vi "Draw Tree Elements.vi"(0 "Decision Tree In":T3, 1 "[user-specified font]":T2, 2 "Width Padding":i32, 3 "Height Padding":i32, 5 "2D Picture in":picture, 7 "Outcome Font":T2, 9 "pen":T1, 11 "Leaf Circle Radius":i32=8) -> (4 "2D Picture out":picture)   [LabVIEW 2025]
uses:
  Types/Decision Tree.ctl
  Types/Sequencing Tree Node.ctl
  Types/Single Cmd Info.ctl
  <vilib>/picture/picture.llb/imagedata.ctl
  <vilib>/Analysis/baseanly.llb/Mean (DBL).vi
  <vilib>/Analysis/NI_AALBase.lvlib
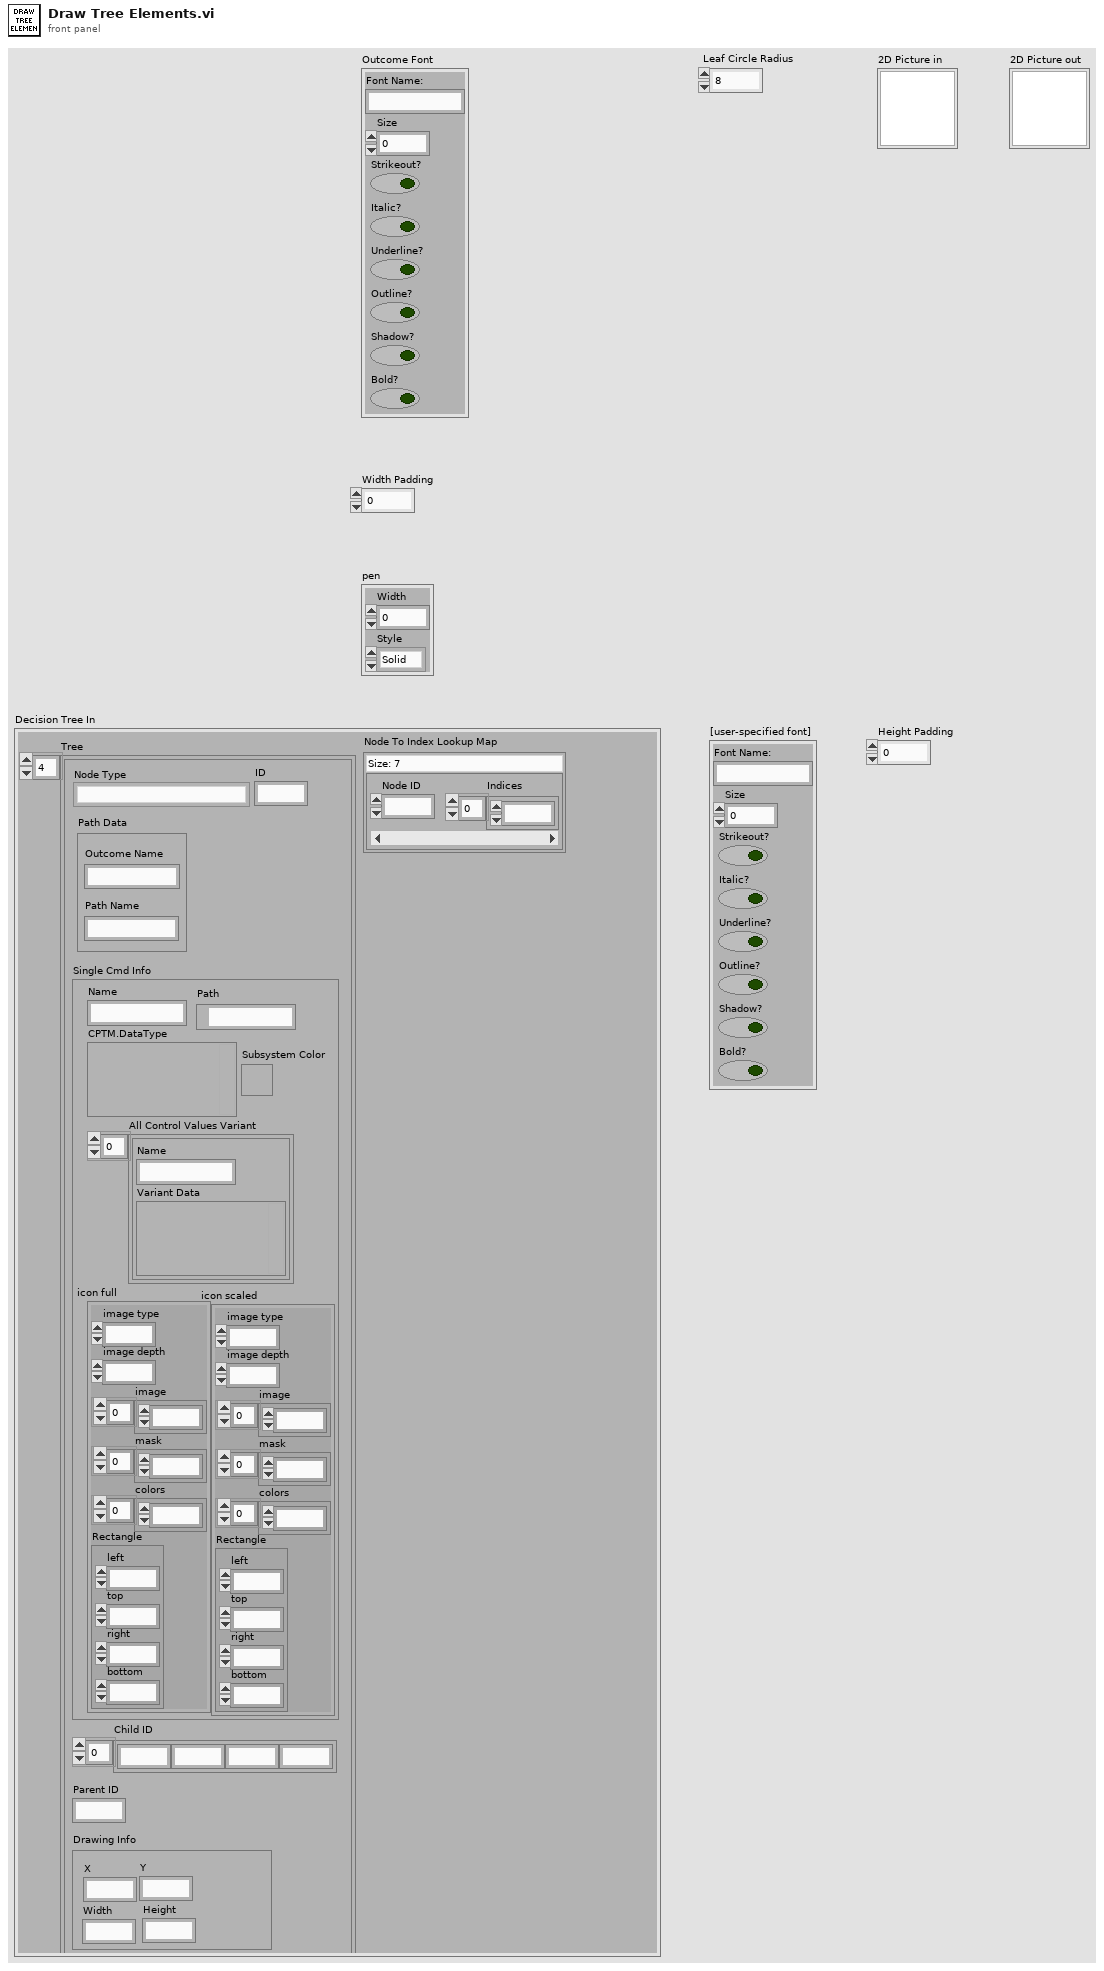
[diagram p1: front panel]
types:
  T1 = cluster{"Width":i16, "Style":enum32{"Solid", "Dash", "Dot", "DashDot", "DashDotDot"}}
  T2 = cluster{"Font Name:":string, "Size":i16, "Strikeout?":bool, "Italic?":bool, "Underline?":bool, "Outline?":bool, "Shadow?":bool, "Bold?":bool}
  T3 = typedef "Decision Tree.ctl" = cluster{"Tree":T4[], "Node To Index Lookup Map":map{i16, i16[]}}
  T4 = typedef "Sequencing Tree Node.ctl" = cluster{"Node Type":enum16{"Path", "Command", "Leaf"}, "ID":i16, "Path Data":cluster{"Path Name":string, "Outcome Name":string}, "Single Cmd Info":T5, "Child ID":i32[], "Parent ID":i32, "Drawing Info":cluster{"X":i32, "Y":i32, "Width":i32, "Height":i32}}
  T5 = typedef "Single Cmd Info.ctl" = cluster{"Name":string, "CPTM.DataType":variant, "All Control Values Variant":cluster{"Name":string, "Variant Data":variant}[], "icon full":T6, "icon scaled":T6, "Path":path, "Subsystem Color":u32}
  T6 = typedef "imagedata.ctl" = cluster{"image type":i32, "image depth":i32, "image":u8[], "mask":u8[], "colors":u32[], "Rectangle":cluster{"left":i16, "top":i16, "right":i16, "bottom":i16}}
  T7 = cluster{"Width":u16, "Style":enum32{"Solid", "Dash", "Dot", "DashDot", "DashDotDot"}}
  T8 = cluster{"horizontal":enum16{"left", "center", "right"}, "vertical":enum16{"top", "center", "bottom"}}
  T9 = enum16{"User-specified Font", "Application Font", "System Font", "Dialog Font"}
  T10 = cluster{"Path Name":string, "Outcome Name":string}
  T11 = cluster{"X":i32, "Y":i32, "Width":i32, "Height":i32}
  T12 = cluster{"left":i16, "top":i16, "right":i16, "bottom":i16}
  T13 = cluster{"[0]":dbl, "[1]":dbl, "[2]":dbl, "[3]":dbl}
  T14 = cluster{"X":dbl, "Y":dbl, "Width":dbl, "Height":dbl}
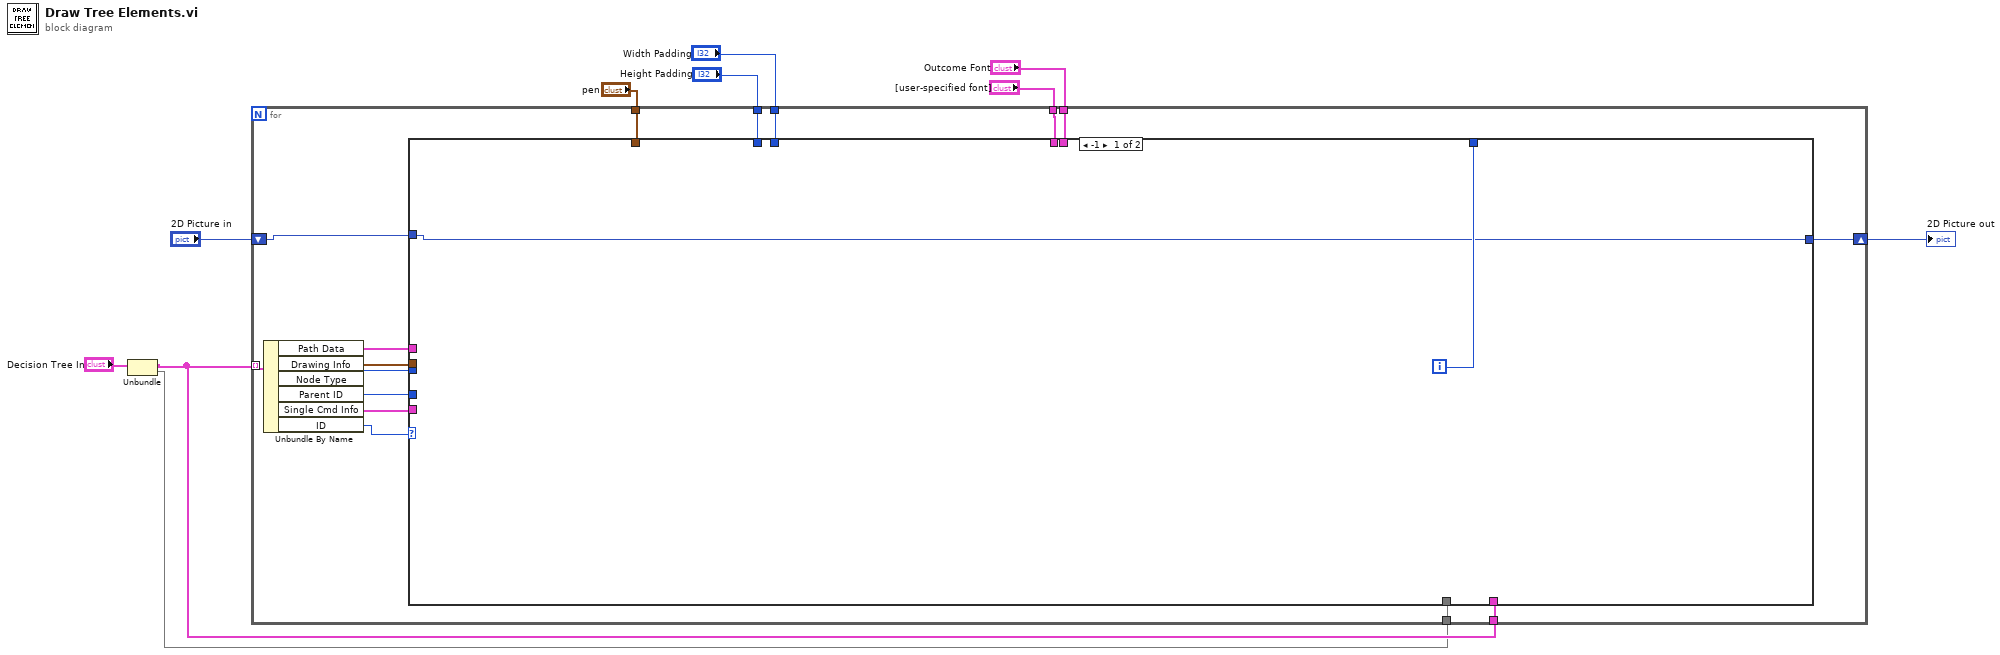
[diagram p0: block diagram]
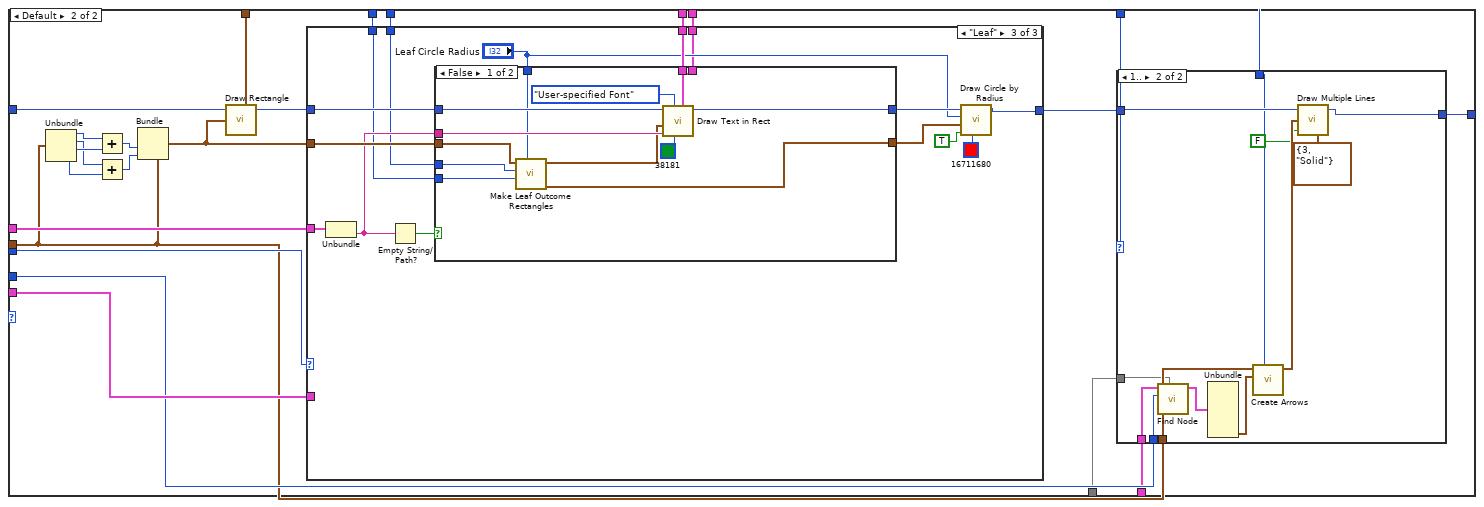
[diagram p2: hidden frame]
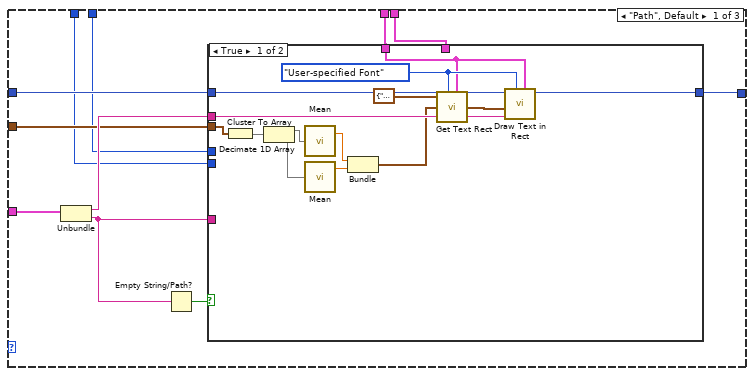
[diagram p4: hidden frame]
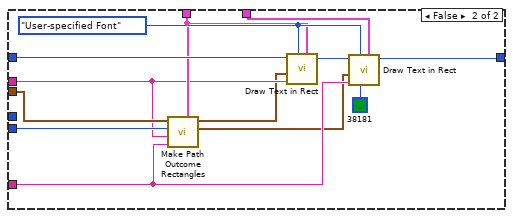
[diagram p5: hidden frame]
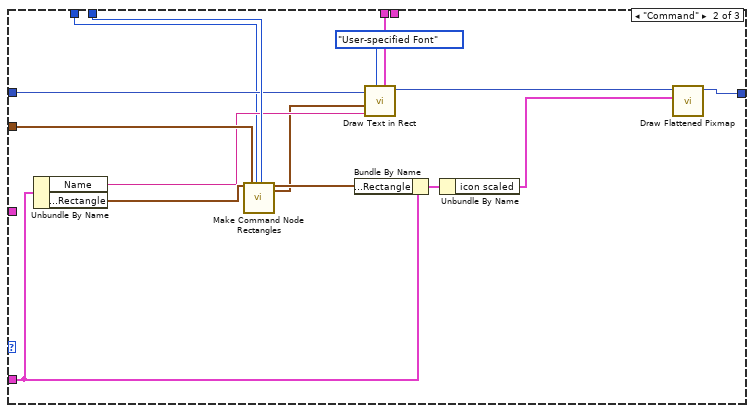
[diagram p6: hidden frame]
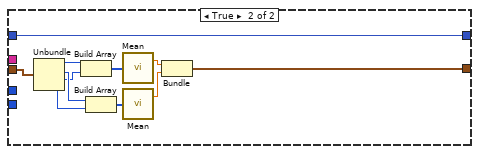
[diagram p7: hidden frame]
diagram:
  n1 = Unbundle("Decision Tree In") -> ("Tree"=w2:T4[], "Node To Index Lookup Map"=w1:map{i16, i16[]})
  n2 = for {
    tunnel: w2 -> [w27] mode=indexing
    shift-right: [w14] -> w8
    shift-left: "2D Picture in" -> [w26]
    tunnel: "pen" -> [w25]
    tunnel: w2 -> [w13]
    tunnel: "Width Padding" -> [w22]
    tunnel: "[user-specified font]" -> [w21]
    tunnel: "Height Padding" -> [w15]
    tunnel: "Outcome Font" -> [w19]
    tunnel: w1 -> [w12]
    i -> [w18]
    n3 = Unbundle By Name(w27) -> ("Path Data"=w20:T10, "Drawing Info"=w16:T11, "Node Type"=w24:enum16{"Path", "Command", "Leaf"}, "Parent ID"=w17:i32, "Single Cmd Info"=w23:T5, "ID"=w11:i16)
    n4 = case shown="-1" w11 {
      tunnel: w26 -> [w28 w52]
      tunnel: w25 -> [_ w51]
      tunnel: w24 -> [_ w44]
      tunnel: w23 -> [_ w42]
      tunnel: w22 -> [_ w41]
      tunnel: w21 -> [_ w40]
      tunnel: w20 -> [_ w39]
      tunnel: w19 -> [_ w38]
      tunnel: w18 -> [_ w36]
      tunnel: w17 -> [_ w35]
      tunnel: w16 -> [_ w34]
      tunnel: w15 -> [_ w32]
      tunnel: [w28 w31] -> w14
      tunnel: w13 -> [_ w30]
      tunnel: w12 -> [_ w29]
      frame -1 {
      }
      frame Default {
        n5 = Unbundle(w34) -> ("X"=w50:i32, "Y"=w48:i32, "Width"=w49:i32, "Height"=w47:i32)
        n6 = Add(x=w50, y=w49) -> (x+y=w46:i32)
        n7 = Add(x=w48, y=w47) -> (x+y=w45:i32)
        n8 = Bundle(cluster=w34, "Width"=w46, "Height"=w45) -> (w33:T11)  [unwired: 2 in]
        n9 = call <vilib>:"Draw Rectangle.vi"("picture"=w52, "rect"=w33, "pen"=w51) -> ("new picture"=w43:picture)  [unwired: 6 in]
        n10 = case shown="\"Leaf\"" w44 {
          tunnel: w43 -> [w75 w107 w127]
          tunnel: w33 -> [w72 w111 w125]
          tunnel: [w70 w105 w130] -> w37
          tunnel: w42 -> [_ w113 _]
          tunnel: w41 -> [w71 w110 w122]
          tunnel: w40 -> [w76 w115 w124]
          tunnel: w39 -> [w74 _ w129]
          tunnel: w32 -> [w69 w104 w120]
          tunnel: w38 -> [w67 _ w119]
          frame "Path", Default {
            n11 = Unbundle(w74) -> ("Path Name"=w73:string, "Outcome Name"=w66:string)
            n12 = Empty String/Path?(string/path=w66) -> (empty?=w68:bool)
            n13 = case shown="True" w68 {
              tunnel: w76 -> [w88 w95]
              tunnel: w75 -> [w90 w103]
              tunnel: w73 -> [w86 w94]
              tunnel: w72 -> [w84 w96]
              tunnel: w71 -> [_ _]
              tunnel: [w85 w100] -> w70
              tunnel: w69 -> [_ w97]
              tunnel: w67 -> [_ w99]
              tunnel: w66 -> [_ w93]
              frame True {
                w89 = T9."User-specified Font" ("desired font(Application)")
                n14 = Cluster To Array(cluster=w84) -> (array=w83:i32[])
                n15 = Decimate 1D Array(w83) -> (w80:i32[], w79:i32[])
                n16 = call-poly <vilib>:"Mean.vi"("X"=w80) -> ("mean"=w82:dbl)  [unwired: 1 out]
                n17 = call-poly <vilib>:"Mean.vi"("X"=w79) -> ("mean"=w81:dbl)  [unwired: 1 out]
                n18 = Bundle("mean"=w82, "mean"=w81) -> (w78:cluster{"mean":dbl, "mean":dbl})  [unwired: 1 in]
                n19 = call <vilib>:"Get Text Rect.vi"("alignment(left, top)"=T8 {"horizontal"=enum."center", "vertical"=enum."center"}, "desired font(Application)"=w89, "origin(0,0)"=w78, "text"=w86, "[user-specified font]"=w88) -> ("rect"=w87:T12)  [unwired: 4 in]
                n20 = call <vilib>:"Draw Text in Rect.vi"("[user-specified font]"=w88, "desired font(Application)"=w89, "text"=w86, "rect"=w87, "picture"=w90) -> ("new picture"=w85:picture)  [unwired: 6 in]
              }
              frame False {
                w102 = T9."User-specified Font" ("desired font(Application)")
                n21 = call "Make Path Outcome Rectangles.vi"("[user-specified font]"=w95, "Outcome Name"=w93, "Path Name"=w94, "Height Padding"=w97, "Drawing Info"=w96) -> ("Outcome Name Rect"=w91:T12, "Path Name Rect"=w92:T12)  [unwired: 5 in]
                n22 = call <vilib>:"Draw Text in Rect.vi"("[user-specified font]"=w95, "desired font(Application)"=w102, "text"=w94, "rect"=w92, "picture"=w103) -> ("new picture"=w101:picture)  [unwired: 6 in]
                n23 = call <vilib>:"Draw Text in Rect.vi"("[user-specified font]"=w99, "text color(black)"=u32 38181, "desired font(Application)"=w102, "text"=w93, "rect"=w91, "picture"=w101) -> ("new picture"=w100:picture)  [unwired: 5 in]
              }
            }
          }
          frame "Command" {
            n24 = Unbundle By Name(w113) -> ("Name"=w109:string, "icon scaled.Rectangle"=w112:T12)
            n25 = call "Make Command Node Rectangles.vi"("Icon Rectangle"=w112, "Node Rectangle"=w111, "Height Padding"=w104, "Width Padding"=w110) -> ("New Icon Rectangle"=w118:T13, "Text Rectangle"=w108:T13)  [unwired: 14 in]
            n26 = Bundle By Name(cluster=w113, "icon scaled.Rectangle"=w118) -> (w117:T5)
            n27 = call <vilib>:"Draw Text in Rect.vi"("[user-specified font]"=w115, "desired font(Application)"=T9."User-specified Font", "text"=w109, "rect"=w108, "picture"=w107) -> ("new picture"=w106:picture)  [unwired: 6 in]
            n28 = Unbundle By Name(w117) -> ("icon scaled"=w116:T6)
            n29 = call <vilib>:"Draw Flattened Pixmap.vi"("image data"=w116, "picture"=w106) -> ("new picture"=w105:picture)  [unwired: 7 in]
          }
          frame "Leaf" {
            n30 = Unbundle(w129) -> ("Outcome Name"=w123:string)  [unwired: 1 out]
            n31 = Empty String/Path?(string/path=w123) -> (empty?=w128:bool)
            n32 = case shown="False" w128 {
              tunnel: [w137 w152] -> w131
              tunnel: w127 -> [w145 w151]
              tunnel: [w142 w151] -> w126
              tunnel: w125 -> [w141 w150]
              tunnel: w124 -> [_ _]
              tunnel: w123 -> [w143 _]
              tunnel: w122 -> [w138 _]
              tunnel: "Leaf Circle Radius" -> [w136 _]
              tunnel: w120 -> [w140 _]
              tunnel: w119 -> [w135 _]
              frame False {
                n33 = call "Make Leaf Outcome Rectangles.vi"("Leaf Circle Radius"=w136, "Height Padding"=w140, "Width Padding"=w138, "Drawing Info in"=w141) -> ("Leaf Circle Center"=w137:cluster{"mean":dbl, dbl}, "Text Rectangle"=w139:T14)  [unwired: 6 in]
                n34 = call <vilib>:"Draw Text in Rect.vi"("[user-specified font]"=w135, "text color(black)"=u32 38181, "desired font(Application)"=T9."User-specified Font", "text"=w143, "rect"=w139, "picture"=w145) -> ("new picture"=w142:picture)  [unwired: 5 in]
              }
              frame True {
                n35 = Unbundle(w150) -> ("X"=w149:i32, "Y"=w148:i32, "Width"=w147:i32, "Height"=w146:i32)
                n36 = Build Array(w149, w147) -> (w156:i32[])
                n37 = Build Array(w148, w146) -> (w155:i32[])
                n38 = call-poly <vilib>:"Mean.vi"("X"=w156) -> ("mean"=w154:dbl)  [unwired: 1 out]
                n39 = call-poly <vilib>:"Mean.vi"("X"=w155) -> ("mean"=w153:dbl)  [unwired: 1 out]
                n40 = Bundle("mean"=w154, "mean"=w153) -> (w152:cluster{"mean":dbl, "mean":dbl})  [unwired: 1 in]
              }
            }
            n41 = call <vilib>:"Draw Circle by Radius.vi"("color(black)"=u32 16711680, "fill?(F)"=TRUE, "pixel center"=w131, "radius"="Leaf Circle Radius", "picture"=w126) -> ("new picture"=w130:picture)  [unwired: 6 in]
          }
        }
        n42 = case shown="1.." w36 {
          tunnel: w37 -> [w53 w65]
          tunnel: [w53 w64] -> w31
          tunnel: w35 -> [_ w56]
          tunnel: w34 -> [_ w60]
          tunnel: w32 -> [_ w58]
          tunnel: w30 -> [_ w55]
          tunnel: w29 -> [_ w54]
          frame 0, Default {
          }
          frame 1.. {
            n43 = call "Find Node.vi"("Node To Index Lookup Map"=w54, "ID"=w56, "Tree"=w55) -> ("Node"=w57:T4)  [unwired: 7 in, 1 out]
            n44 = Unbundle(w57) -> ("Drawing Info"=w59:T11)  [unwired: 6 out]
            n45 = call "Create Arrows.vi"("Height Padding"=w58, "Drawing Info Parent"=w59, "Drawing Info Child"=w60) -> ("Arrows"=w62:cluster{dbl, dbl}[])  [unwired: 8 in]
            n46 = call <vilib>:"Draw Multiple Lines.vi"("picture"=w65, "line endpoints"=w62, "fill?(F)"=FALSE, "pen"=T7 {"Width"=3, "Style"=enum."Solid"}) -> ("new picture"=w64:picture)  [unwired: 5 in]
          }
        }
      }
    }
  }
  "2D Picture out" <- w8
